vi "Write Expired.vi"(8 "error in (no error)":errorcluster, 10 "Expired?":bool, 11 "AcknowledgeMsg in":refnum<class "CS++AcknowledgeMsg.lvclass">) -> (0 "error out":errorcluster, 3 "AcknowledgeMsg out":refnum<class "CS++AcknowledgeMsg.lvclass">)   [LabVIEW 2015, in "CS++AcknowledgeMsg.lvlib" / "CS++AcknowledgeMsg.lvclass"]
uses:
  CS++AcknowledgeMsg.lvclass
  CS++AcknowledgeMsg.lvclass/CS++AcknowledgeMsg.ctl
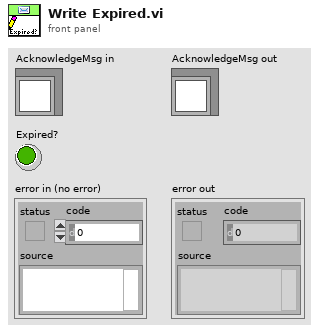
[diagram p1: front panel]
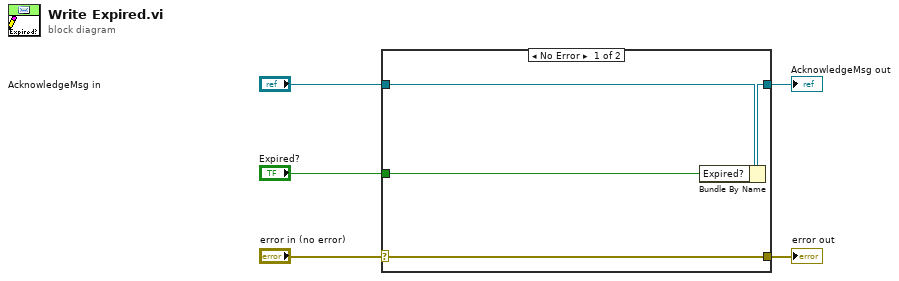
[diagram p0: block diagram]
diagram:
  n1 = case shown="No Error" "error in (no error)" {
    selector: "error in (no error)" -> [w9 w10]
    tunnel: [w9 w10] -> w4
    tunnel: [w7 w11] -> w2
    tunnel: "AcknowledgeMsg in" -> [w8 w11]
    tunnel: "Expired?" -> [w6 _]
    frame No Error {
      n2 = Bundle By Name(cluster=w8, "Expired?"=w6) -> (w7:refnum<class "CS++AcknowledgeMsg.lvclass">)
    }
    frame Error {
    }
  }
  "error out" <- w4
  "AcknowledgeMsg out" <- w2
